vi "lock_semaphore.vi"(8 "error in (no error)":errorcluster, 11 "PrepLineObject in":refnum<class "PrepLineObject.lvclass">) -> (0 "error out":errorcluster, 3 "PrepLineObject out":refnum<class "PrepLineObject.lvclass">)   [LabVIEW 2018, in "PrepLineObject.lvclass"]
doc: "locks the semaphore for this pbject in order to restrict access to one process only"
uses:
  PrepLineObject.lvclass
  PrepLineObject.lvclass/PrepLineObject.ctl
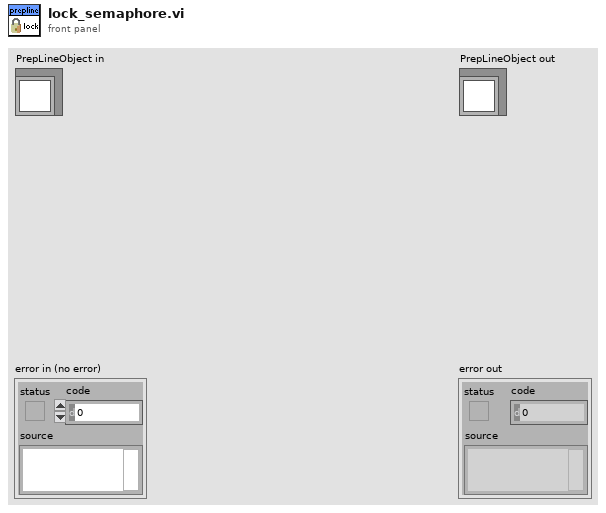
[diagram p1: front panel]
types:
  T1 = typedef "Semaphore RefNum" = refnum<k1>
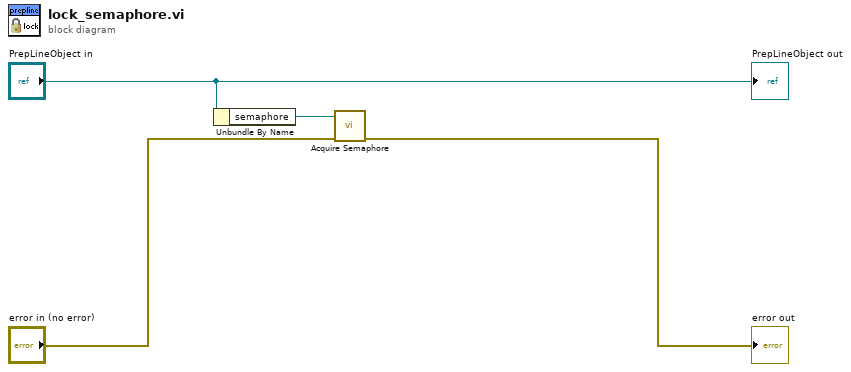
[diagram p0: block diagram]
diagram:
  n1 = Unbundle By Name("PrepLineObject in") -> ("semaphore"=w1:T1)
  n2 = call <vilib>:"Acquire Semaphore.vi"("error in (no error)"="error in (no error)", "semaphore"=w1) -> ("error out"=→"error out":errorcluster)  [unwired: 3 in, 2 out]
  "PrepLineObject out" <- "PrepLineObject in"
